vi "LAB-IQ Main.vi"() -> ()   [LabVIEW 2025]
doc: "This template is for the Queued Message Handler design pattern.\n\nThe Event Handling Loop generates messages based on user interface actions.\n\nThe Message Handling Loop processes messages generated by the Event Handling Loop, or by other messages. The messages are string values, so new messages can be added easily to the Message Cases case structure in the Message Handling Loop. Each message cluster can also provide an optional value for Message Data, which is a variant that can be converted to whatever message-specific data is required."
uses:
  controls/LAB-IQ UI Data.ctl
  support/Message Queue/Enqueue Message (Single).vi
  <vilib>/Utility/error.llb/Error Cluster From Error Code.vi
  <vilib>/ErrorRing/Error Ring.xnode
  support/Message Queue/LAB-IQ Message Queue.lvlib
  support/User Event - Stop/LAB-IQ User Event - Stop.lvlib
panel:
  out "Display <Replace Me>":string
  in  "Do Something Else <Replace Me>":bool
  in  "Do Something <Replace Me>":bool
  in  "Exit":bool
  # "These controls have associated \"Value Changed\" events configured in the Event Structure on the diagram.\n\nReplace them (and reconfigure the Event Structure) with the controls you need for your application."
  # "This template is for the Queued Message Handler design pattern.\n\nSee the block diagram for more information on how to use this template."
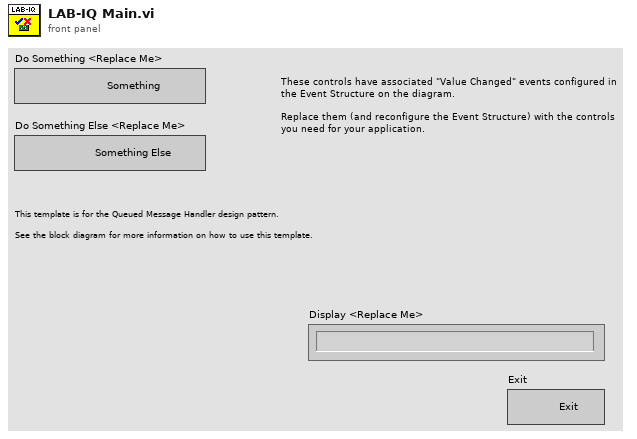
[diagram p1: front panel]
types:
  T1 = typedef "LAB-IQ UI Data.ctl" = cluster{"Main Home Screen":cluster{"GUI":refnum<vi>, "Platform Settings":refnum<vi>, "Configure":refnum<vi>, "Home":refnum<vi>, "EXIT":refnum<vi>, "service 2":refnum<vi>, "MainPage":refnum<vi>}, "Platform Settings":cluster{"mm/s  Surge":refnum<vi>, "Update Surge Speed":refnum<vi>, "Drive Error":refnum<vi>, "Disable Axis Jog Soft Limits":refnum<vi>, "mm/s  Sway":refnum<vi>, "Sway and Surge COM Status":refnum<vi>, "Heave COM Status":refnum<vi>, "Enable Platform":refnum<vi>, "Surge Forward Main":refnum<vi>, "Sway Right Main":refnum<vi>, "Sway Left Main":refnum<vi>, "Heave Down Main":refnum<vi>, "Heave Up main":refnum<vi>, "Update Sway Speed":refnum<vi>, "Update Heave Speed":refnum<vi>, "mm/s Heave":refnum<vi>, "mm/sec":refnum<vi>, "mm":refnum<vi>}, "Analysis Screen":cluster{"Analysis Home":refnum<vi>, "Surface Analysis":refnum<vi>, "Imaging":refnum<vi>, "Image Analysis":refnum<vi>, "Post Analysis":refnum<vi>}, "Config Screen":cluster{"Select Load Head":refnum<vi>, "Notes :":refnum<vi>, "FILE":refnum<vi>, "Sample ID :":refnum<vi>, "Operator ID :":refnum<vi>, "Operator Name :":refnum<vi>, "Auto":refnum<vi>}}
  T2 = typedef "LAB-IQ Message Queue.lvlib/All Message Queues.ctl" = cluster{"UI":refnum<queue>}
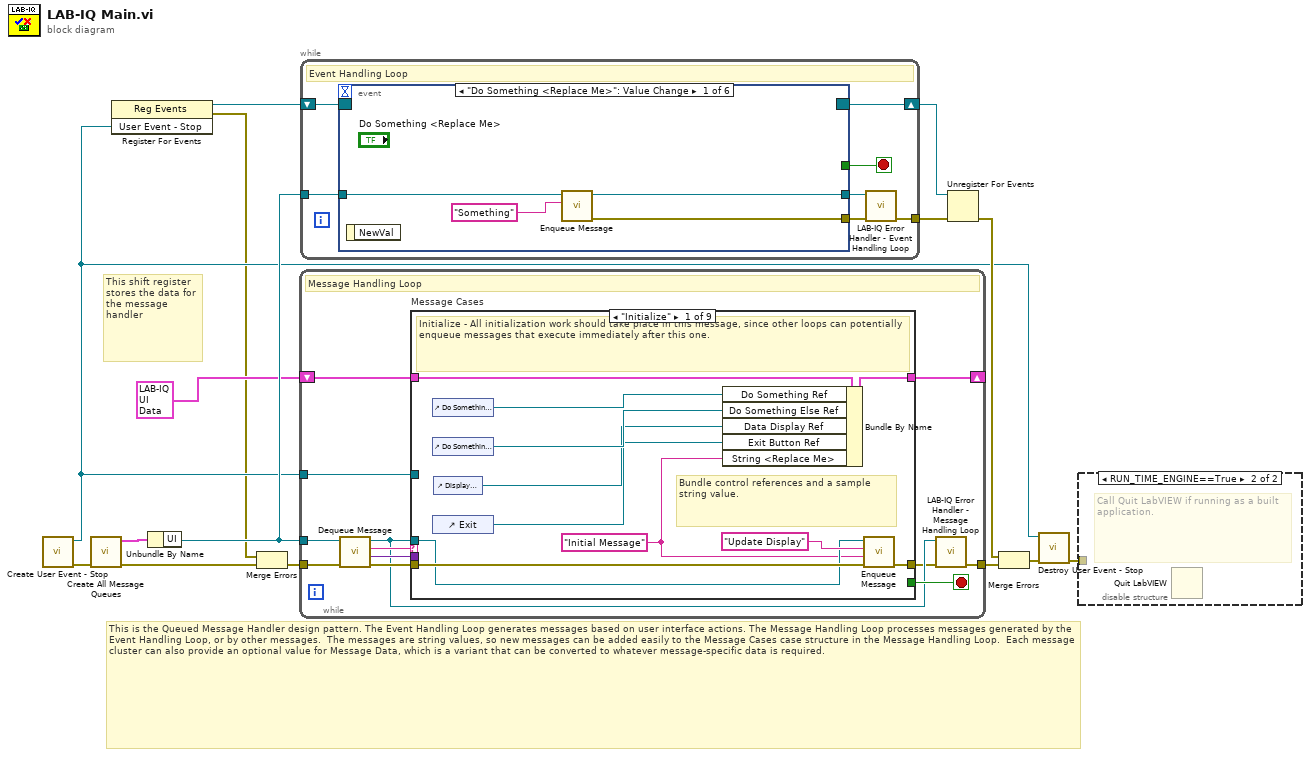
[diagram p0: block diagram]
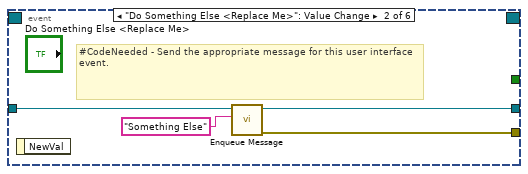
[diagram p3: hidden frame]
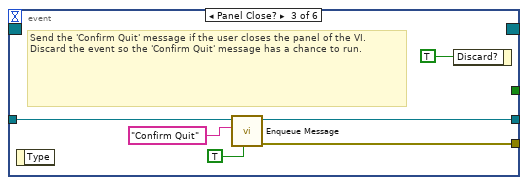
[diagram p4: hidden frame]
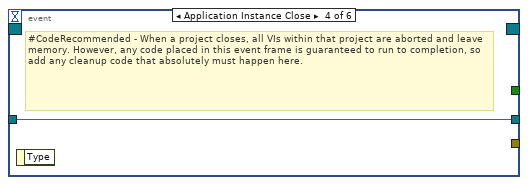
[diagram p5: hidden frame]
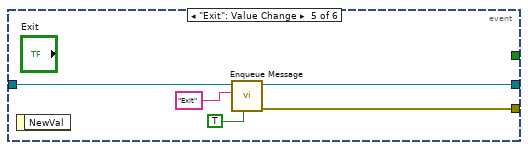
[diagram p6: hidden frame]
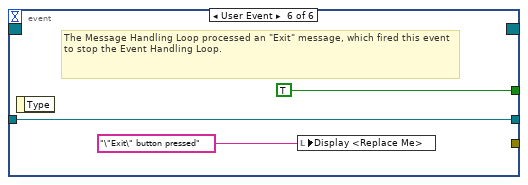
[diagram p7: hidden frame]
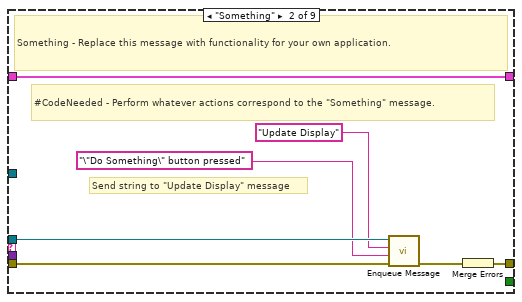
[diagram p8: hidden frame]
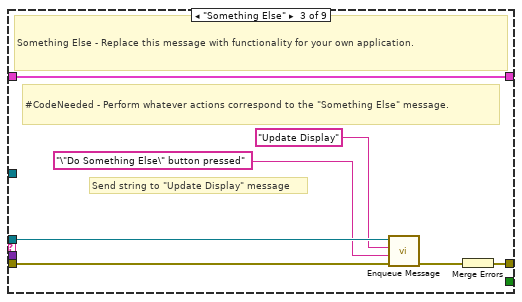
[diagram p9: hidden frame]
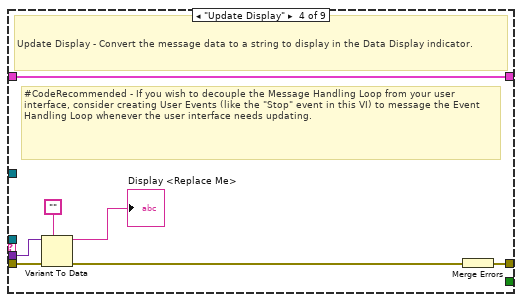
[diagram p10: hidden frame]
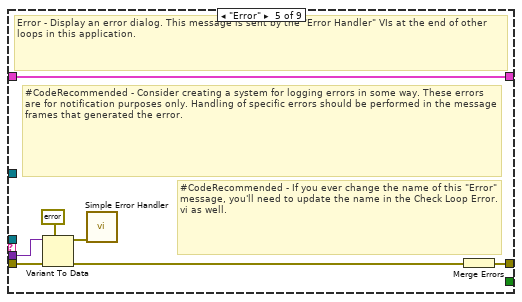
[diagram p11: hidden frame]
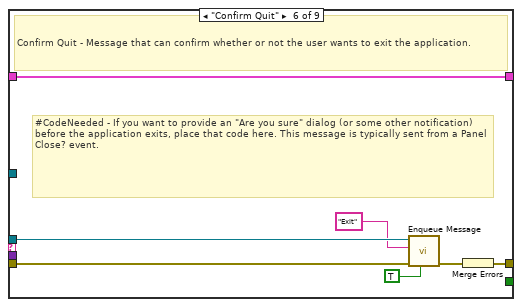
[diagram p12: hidden frame]
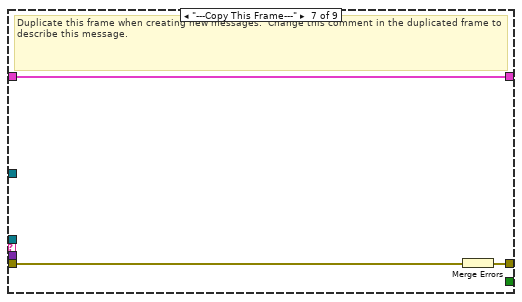
[diagram p13: hidden frame]
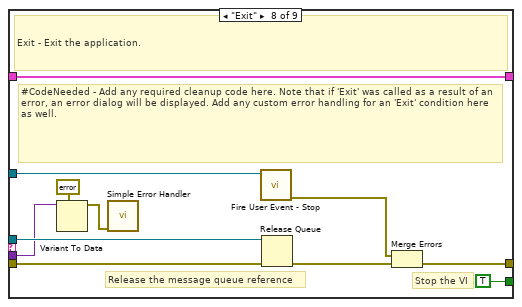
[diagram p14: hidden frame]
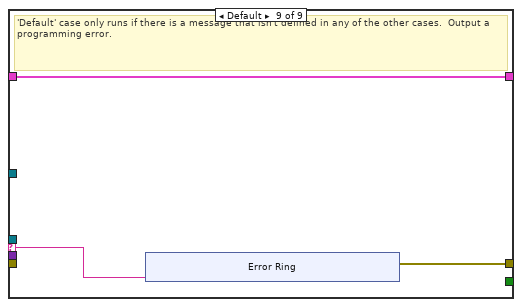
[diagram p15: hidden frame]
diagram:
  # "This is the Queued Message Handler design pattern. The Event Handling Loop generates messages based on user interface actions. The Message Handling Loop processes messages generated by the Event Handling Loop, or by other messages.  The messages are string values, so new messages can be added easily to the Message Cases case structure in the Message Handling Loop.  Each message cluster can also provide an optional value for Message Data, which is a variant that can be converted to whatever message-specific data is required."
  # "This shift register stores the data for the message handler"
  n1 = call "Create User Event - Stop.vi"() -> ("error out"=w11:errorcluster, "User Event - Stop"=w3:refnum<user-event>)  [unwired: 10 in]
  n2 = call "Create All Message Queues.vi"("error in (no error)"=w11) -> ("error out"=w15:errorcluster, "Message Queues out"=w14:T2)  [unwired: 9 in]
  n3 = register-events(w3) -> (reference out=w4:refnum<event-registration>, error out=w1:errorcluster)  [unwired: 2 in]
  n4 = Unbundle By Name(w14) -> ("UI"=w12:refnum<queue>)
  n5 = Merge Errors(w1, w15) -> (w2:errorcluster)
  n6 = while {
    tunnel: w12 -> [w19]
    shift-right: [w26] -> _
    shift-left: T1 {"Main Home Screen"={"GUI"=refnum, "Platform Settings"=refnum, "Configure"=refnum, "Home"=refnum, "EXIT"=refnum, "service 2"=refnum, "MainPage"=refnum}, "Platform Settings"={"mm/s  Surge"=refnum, "Update Surge Speed"=refnum, "Drive Error"=refnum, "Disable Axis Jog Soft Limits"=refnum, "mm/s  Sway"=refnum, "Sway and Surge COM Status"=refnum, "Heave COM Status"=refnum, "Enable Platform"=refnum, "Surge Forward Main"=refnum, "Sway Right Main"=refnum, "Sway Left Main"=refnum, "Heave Down Main"=refnum, "Heave Up main"=refnum, "Update Sway Speed"=refnum, "Update Heave Speed"=refnum, "mm/s Heave"=refnum, "mm/sec"=refnum, "mm"=refnum}, "Analysis Screen"={"Analysis Home"=refnum, "Surface Analysis"=refnum, "Imaging"=refnum, "Image Analysis"=refnum, "Post Analysis"=refnum}, "Config Screen"={"Select Load Head"=refnum, "Notes :"=refnum, "FILE"=refnum, "Sample ID :"=refnum, "Operator ID :"=refnum, "Operator Name :"=refnum, "Auto"=refnum}} ("Data Cluster") -> [w27]
    tunnel: w3 -> [w24]
    tunnel: w2 -> [w23]
    tunnel: [w17] -> w13
    stop <- w25 stop-if-true
    # "Message Handling Loop"
    n7 = call "Dequeue Message.vi"("error in (no error)"=w23, "Message Queue"=w19) -> ("error out"=w22:errorcluster, "Message Data"=w20:variant, "Message"=w21:string, "dup Message Queue"=w18:refnum<queue>)  [unwired: 6 in]
    n8 = case "Message Cases" shown="\"Initialize\"" w21 {
      selector: w21 -> [_ _ _ _ _ _ _ _ w88]
      tunnel: w18 -> [w29 w41 w48 _ _ w69 _ w87 _]
      tunnel: w22 -> [w37 w43 w50 w57 w66 w73 w76 w80 _]
      tunnel: [w38 w44 w51 w58 w60 w71 w74 w83 w89] -> w16
      tunnel: w27 -> [w36 w45 w52 w59 w65 w72 w75 w86 w90]
      tunnel: [w35 w45 w52 w59 w65 w72 w75 w86 w90] -> w26
      tunnel: [_ _ _ _ _ _ _ TRUE _] -> w25
      tunnel: w20 -> [_ _ _ w56 w64 _ _ w77 _]
      tunnel: w24 -> [_ _ _ _ _ _ _ w82 _]
      frame "Initialize" {
        w28 = "Initial Message" ("Initial Message")
        # "Bundle control references and a sample string value."
        # "Initialize - All initialization work should take place in this message, since other loops can potentially enqueue messages that execute immediately after this one."
        n9 = control-ref of="Do Something <Replace Me>"() -> (w34:refnum<vi>)
        n10 = control-ref of="Do Something Else <Replace Me>"() -> (w33:refnum<vi>)
        n11 = control-ref of="Exit"() -> (w31:refnum<vi>)
        n12 = control-ref of="Display <Replace Me>"() -> (w32:refnum<vi>)
        n13 = Bundle By Name(cluster=w36, "Do Something Ref"=w34, "Do Something Else Ref"=w33, "Data Display Ref"=w32, "Exit Button Ref"=w31, "String <Replace Me>"=w28) -> (w35:T1)
        n14 = call-poly "Enqueue Message.vi"("error in (no error)"=w37, "Message Data"=w28, "Message"="Update Display", "Message Queue"=w29) -> ("error out"=w38:errorcluster)  [unwired: 6 in, 1 out]
      }
      frame "Something" {
        # "Send string to \"Update Display\" message"
        # "#CodeNeeded - Perform whatever actions correspond to the \"Something\" message."
        # "Something - Replace this message with functionality for your own application."
        n15 = call-poly "Enqueue Message.vi"("error in (no error)"=w43, "Message Data"="\"Do Something\" button pressed" ("\"Do Something\" button pressed"), "Message"="Update Display", "Message Queue"=w41) -> ("error out"=w42:errorcluster)  [unwired: 6 in, 1 out]
        n16 = Merge Errors(w42) -> (w44:errorcluster)
      }
      frame "Something Else" {
        # "Send string to \"Update Display\" message"
        # "#CodeNeeded - Perform whatever actions correspond to the \"Something Else\" message."
        # "Something Else - Replace this message with functionality for your own application."
        n17 = call-poly "Enqueue Message.vi"("error in (no error)"=w50, "Message Data"="\"Do Something Else\" button pressed" ("\"Do Something Else\" button pressed"), "Message"="Update Display", "Message Queue"=w48) -> ("error out"=w49:errorcluster)  [unwired: 6 in, 1 out]
        n18 = Merge Errors(w49) -> (w51:errorcluster)
      }
      frame "Update Display" {
        # "#CodeRecommended - If you wish to decouple the Message Handling Loop from your user interface, consider creating User Events (like the \"Stop\" event in this VI) to message the Event Handling Loop whenever the user interface needs updating."
        # "Update Display - Convert the message data to a string to display in the Data Display indicator."
        n19 = Variant To Data(error in=w57, type="", Variant=w56) -> (data=→"Display <Replace Me>":string, error out=w54:errorcluster)
        n20 = Merge Errors(w54) -> (w58:errorcluster)
      }
      frame "Error" {
        # "#CodeRecommended - If you ever change the name of this \"Error\" message, you'll need to update the name in the Check Loop Error.vi as well."
        # "#CodeRecommended - Consider creating a system for logging errors in some way. These errors are for notification purposes only. Handling of specific errors should be performed in the message frames that generated the error."
        # "Error - Display an error dialog. This message is sent by the \"Error Handler\" VIs at the end of other loops in this application."
        n21 = Variant To Data(error in=w66, type=errorcluster {"status"=FALSE, "code"=0, "source"=""} ("error constant"), Variant=w64) -> (data=w62:errorcluster, error out=w61:errorcluster)
        n22 = call <vilib>:"Simple Error Handler.vi"("error in (no error)"=w62) -> ()  [unwired: 4 in, 5 out]
        n23 = Merge Errors(w61) -> (w60:errorcluster)
      }
      frame "Confirm Quit" {
        # "#CodeNeeded - If you want to provide an \"Are you sure\" dialog (or some other notification) before the application exits, place that code here. This message is typically sent from a Panel Close? event."
        # "Confirm Quit - Message that can confirm whether or not the user wants to exit the application."
        n24 = call-poly "Enqueue Message.vi"("Priority Message? (F)"=TRUE, "error in (no error)"=w73, "Message"="Exit", "Message Queue"=w69) -> ("error out"=w70:errorcluster)  [unwired: 6 in, 1 out]
        n25 = Merge Errors(w70) -> (w71:errorcluster)
      }
      frame "---Copy This Frame---" {
        # "Duplicate this frame when creating new messages.  Change this comment in the duplicated frame to describe this message."
        n26 = Merge Errors(w76) -> (w74:errorcluster)
      }
      frame "Exit" {
        # "Stop the VI"
        # "Release the message queue reference"
        # "#CodeNeeded - Add any required cleanup code here. Note that if 'Exit' was called as a result of an error, an error dialog will be displayed. Add any custom error handling for an 'Exit' condition here as well."
        # "Exit - Exit the application."
        n27 = Variant To Data(type=errorcluster {"status"=FALSE, "code"=0, "source"=""} ("error constant"), Variant=w77) -> (data=w78:errorcluster)  [unwired: 1 in, 1 out]
        n28 = call <vilib>:"Simple Error Handler.vi"("error in (no error)"=w78) -> ()  [unwired: 4 in, 5 out]
        n29 = call "Fire User Event - Stop.vi"("User Event - Stop"=w82) -> ("error out"=w81:errorcluster)  [unwired: 10 in]
        n30 = Release Queue(queue=w87, error in (no error)=w80) -> (error out=w84:errorcluster)  [unwired: 1 in, 2 out]
        n31 = Merge Errors(w81, w84) -> (w83:errorcluster)
      }
      frame Default {
        # "'Default' case only runs if there is a message that isn't defined in any of the other cases.  Output a programming error."
        n32 = xnode "Error Ring"("parameter 0"=w88) -> ("error out"=w89:errorcluster)
      }
    }
    n33 = call "LAB-IQ Error Handler - Message Handling Loop.vi"("error in (no error)"=w16, "Message Queue"=w18) -> ("dup error in"=w17:errorcluster)  [unwired: 8 in, 1 out]
  }
  n34 = while {
    tunnel: w12 -> [w104]
    shift-right: [w102] -> w8
    shift-left: w4 -> [w103]
    tunnel: [w98] -> w5
    stop <- w100 stop-if-true
    # "Event Handling Loop"
    n35 = event shown="[0] \"Do Something <Replace Me>\": Value Change" {
      selector: w103 -> [_ _ _ _ _ _]
      dyn-events: [_ _ _ _ _ _] -> w102
      timeout: _ -> [_ _ _ _ _ _]
      tunnel: [_ _ _ _ _ TRUE ("Discard?")] -> w100
      tunnel: w104 -> [w108 w112 w117 w119 w124 w127]
      tunnel: [w105 w109 w116 _ w123 _] -> w101
      tunnel: [w107 w111 w115 w119 w122 w127] -> w99
      event "Do Something <Replace Me>": Value Change {
        n36 = event-data() -> ()  [unwired: 1 in, 1 out]
        n37 = call-poly "Enqueue Message.vi"("Message"="Something", "Message Queue"=w108) -> ("error out"=w105:errorcluster, "dup Message Queue"=w107:refnum<queue>)  [unwired: 8 in]
      }
      event "Do Something Else <Replace Me>": Value Change {
        # "#CodeNeeded - Send the appropriate message for this user interface event."
        n38 = event-data() -> ()  [unwired: 1 in, 1 out]
        n39 = call-poly "Enqueue Message.vi"("Message"="Something Else", "Message Queue"=w112) -> ("error out"=w109:errorcluster, "dup Message Queue"=w111:refnum<queue>)  [unwired: 8 in]
      }
      event Panel Close? {
        # "Send the 'Confirm Quit' message if the user closes the panel of the VI. Discard the event so the 'Confirm Quit' message has a chance to run."
        n40 = event-data() -> ()  [unwired: 1 in, 1 out]
        n41 = call-poly "Enqueue Message.vi"("Priority Message? (F)"=TRUE, "Message"="Confirm Quit", "Message Queue"=w117) -> ("error out"=w116:errorcluster, "dup Message Queue"=w115:refnum<queue>)  [unwired: 7 in]
        n42 = event-data("Discard?"=TRUE) -> ()  [unwired: 1 in, 1 out]
      }
      event Application Instance Close {
        # "#CodeRecommended - When a project closes, all VIs within that project are aborted and leave memory. However, any code placed in this event frame is guaranteed to run to completion, so add any cleanup code that absolutely must happen here."
        n43 = event-data() -> ()  [unwired: 1 in, 1 out]
      }
      event "Exit": Value Change {
        n44 = event-data() -> ()  [unwired: 1 in, 1 out]
        n45 = call-poly "Enqueue Message.vi"("Priority Message? (F)"=TRUE, "Message"="Exit", "Message Queue"=w124) -> ("error out"=w123:errorcluster, "dup Message Queue"=w122:refnum<queue>)  [unwired: 7 in]
      }
      event User Event {
        # "The Message Handling Loop processed an \"Exit\" message, which fired this event to stop the Event Handling Loop."
        n46 = event-data() -> ()  [unwired: 1 in, 1 out]
        n47 = local write "Display <Replace Me>"("\"Exit\" button pressed" ("VI Stopped")) -> ()
      }
    }
    n48 = call "LAB-IQ Error Handler - Event Handling Loop.vi"("error in (no error)"=w101, "Message Queue"=w99) -> ("dup error in"=w98:errorcluster)  [unwired: 8 in, 1 out]
  }
  n49 = Unregister For Events(event registration refnum=w8, error in=w5) -> (error out=w9:errorcluster)
  n50 = Merge Errors(w9, w13) -> (w10:errorcluster)
  n51 = call "Destroy User Event - Stop.vi"("error in (no error)"=w10, "User Event - Stop"=w3) -> ("error out"=w6:errorcluster)  [unwired: 9 in]
  n52 = disable-structure shown="RUN_TIME_ENGINE==True" {
    disable-tunnel: w6 -> [_ _]
    frame condition #0 (active) {
    }
    frame condition #1 {
      # "Call Quit LabVIEW if running as a built application."
      n53 = Quit LabVIEW() -> ()  [unwired: 1 in]
    }
  }
